vi "set_zoom_from_xml.vi"(8 "error in (no error)":errorcluster, 10 "XML string":string, 11 "TrajectoryMH100122AODRAPS in":refnum<class "TrajectoryMH100122AODRAPS.lvclass">) -> (0 "error out":errorcluster, 3 "TrajectoryMH100122AODRAPS out":refnum<class "TrajectoryMH100122AODRAPS.lvclass">)   [LabVIEW 2010, in "TrajectoryMH100122AODRAPS.lvclass"]
uses:
  TrajectoryMH100122AODRAPS.lvclass
  common/classes/XMLElement/XMLElement/XMLElement.lvclass
  TrajectoryMH100122AODRAPS.lvclass/TrajectoryMH100122AODRAPS.ctl
  common/classes/ErrorController/ErrorController/class_data.vi
  common/classes/ErrorController/ErrorController/ErrorController.lvclass
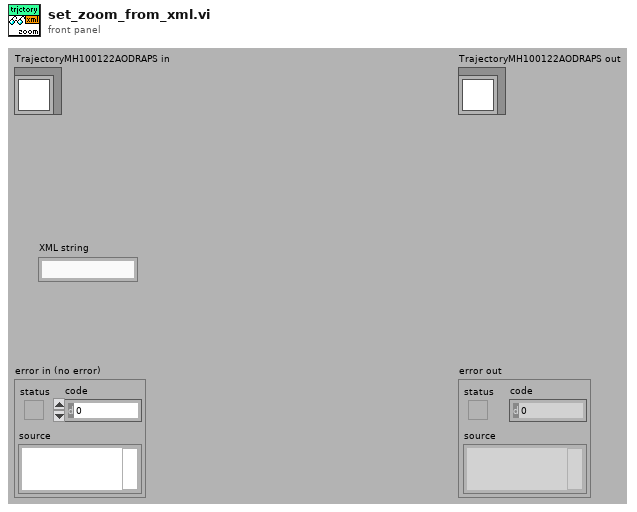
[diagram p1: front panel]
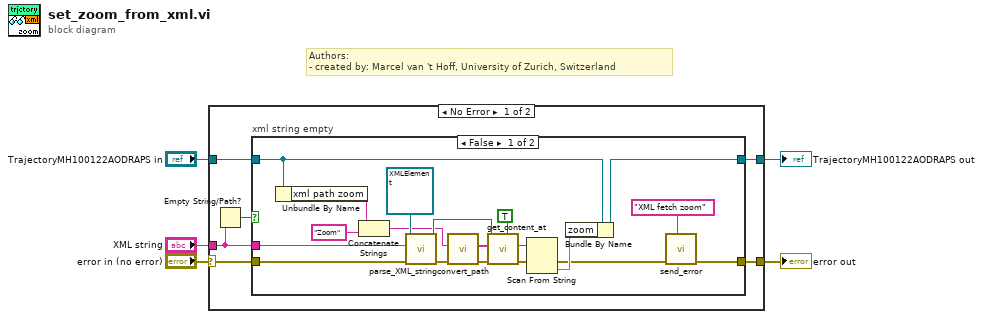
[diagram p0: block diagram]
diagram:
  # "Authors: \n- created by: Marcel van 't Hoff, University of Zurich, Switzerland"
  n1 = case shown="No Error" "error in (no error)" {
    selector: "error in (no error)" -> [w9 w34]
    tunnel: [w8 w34] -> w4
    tunnel: [w10 w33] -> w2
    tunnel: "TrajectoryMH100122AODRAPS in" -> [w11 w33]
    tunnel: "XML string" -> [w7 _]
    frame No Error {
      n2 = Empty String/Path?(string/path=w7) -> (empty?=w6:bool)
      n3 = case "xml string empty" shown="False" w6 {
        tunnel: w11 -> [w19 w32]
        tunnel: [w18 w32] -> w10
        tunnel: w9 -> [w17 w31]
        tunnel: [w15 w31] -> w8
        tunnel: w7 -> [w12 _]
        frame False {
          n4 = Unbundle By Name(w19) -> ("xml path zoom"=w22:string)
          n5 = Concatenate Strings(w22, "Zoom" ("string")) -> (w13:string)
          n6 = call "parse_XML_string.vi"("error in (no error)"=w17, "XML string"=w12, "Element in"=refnum<class "XMLElement.lvclass"> refnum ("XMLElement.lvclass")) -> ("error out"=w28:errorcluster, "Element out"=w27:refnum<class "XMLElement.lvclass">)  [unwired: 6 in, 1 out]
          n7 = call "convert_path.vi"("error in (no error)"=w28, "xpath in"=w13) -> ("error out"=w29:errorcluster, "key array out"=w30:string[])  [unwired: 7 in, 1 out]
          n8 = call "get_content_at.vi"("ignore IDs"=TRUE, "error in (no error)"=w29, "key chain"=w30, "Element in"=w27) -> ("error out"=w25:errorcluster, "string"=w26:string)  [unwired: 4 in, 2 out]
          n9 = Scan From String(input string=w26, error in=w25) -> (error out=w16:errorcluster, output 1=w20:dbl)  [unwired: 3 in, 2 out]
          n10 = Bundle By Name(cluster=w19, "zoom"=w20) -> (w18:refnum<class "TrajectoryMH100122AODRAPS.lvclass">)
          n11 = call "send_error.vi"("additional message"="XML fetch zoom", "error in (no error)"=w16) -> ("error out"=w15:errorcluster)  [unwired: 9 in]
        }
        frame True {
        }
      }
    }
    frame Error {
    }
  }
  "error out" <- w4
  "TrajectoryMH100122AODRAPS out" <- w2
